vi "sub_DSP_TriangInterpolationFilter.vi"(9 "Desired Len":i32, 10 "X":cdb[](array[numeric]), 11 "Interpolation factor":i32) -> (2 "Interpolated X":cdb[](array[numeric]))   [LabVIEW 2012]
uses:
  <vilib>/Analysis/2dsp.llb/1D Convolution (DBL).vi
  <vilib>/Analysis/2dsp.llb/Upsample (CDB).vi
  <vilib>/Analysis/2dsp.llb/1D Convolution (CDB).vi
  <vilib>/Analysis/NI_AALPro.lvlib
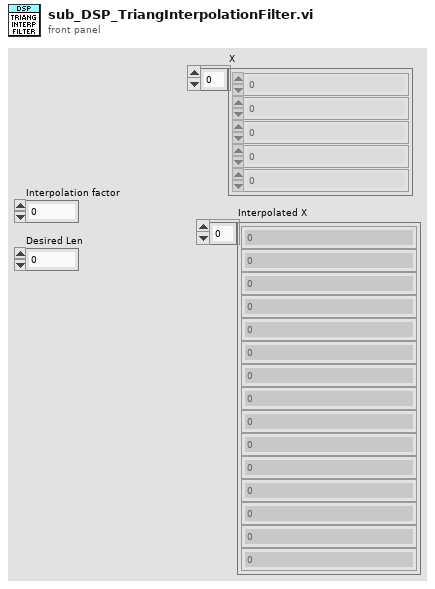
[diagram p1: front panel]
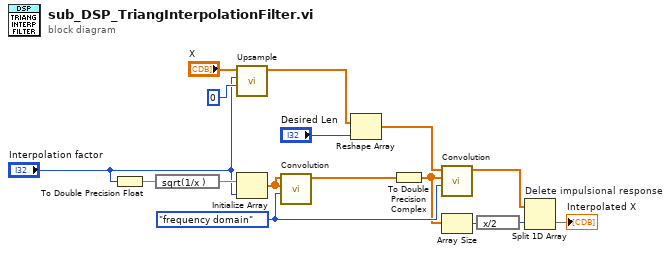
[diagram p0: block diagram]
diagram:
  w6 = enum32{"direct", "frequency domain"}."frequency domain" ("algorithm")
  n1 = To Double Precision Float(number="Interpolation factor") -> (double precision float=w16:dbl)
  n2 = expression code="sqrt(1/x )"(w16) -> (w15:dbl)
  n3 = call-poly <vilib>:"Upsample.vi"("leading zeros"=0 ("upsampling factor"), "upsampling factor"="Interpolation factor", "X"="X") -> ("Upsampled Array"=w11:cdb[])  [unwired: 7 in, 1 out]
  n4 = Initialize Array(w15, "Interpolation factor") -> (w14:dbl[])
  n5 = call-poly <vilib>:"Convolution.vi"("algorithm"=w6, "Y"=w14, "X"=w14) -> ("X * Y"=w7:dbl[])  [unwired: 7 in, 1 out]
  n6 = Reshape Array "Reshape Array"(w11, "Desired Len") -> (w8:cdb[])
  n7 = To Double Precision Complex(1:w7) -> (0:w3:cdb[])
  n8 = call-poly <vilib>:"Convolution.vi"("algorithm"=w6, "Y"=w3, "X"=w8) -> ("X * Y"=w5:cdb[])  [unwired: 7 in, 1 out]
  n9 = Array Size(array=w3) -> (size(s)=w2:i32)
  n10 = expression code="x/2"(w2) -> (w1:i32)
  n11 = Split 1D Array "Delete impulsional response"(array=w5, index=w1) -> (second subarray=→"Interpolated X":cdb[])  [unwired: 1 out]
